vi "Set Direct Sampling.vi"(8 "error in (no error)":errorcluster, 10 "Direct Sampling State":T1, 11 "RTL-SDR in":refnum<class "RTL-SDR.lvclass">) -> (0 "error out":errorcluster, 1 "function return":i32, 3 "RTL-SDR out":refnum<class "RTL-SDR.lvclass">)   [LabVIEW 2015, in "RTL-SDR.lvclass"]
uses:
  RTL-SDR.lvclass
  TypeDef/Direct Sampling States.ctl
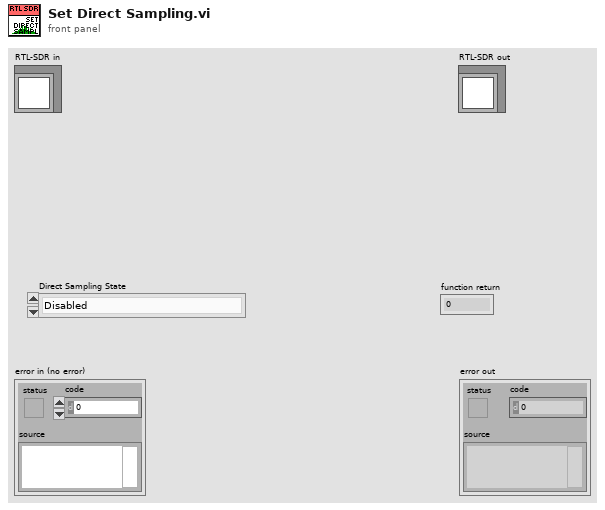
[diagram p1: front panel]
types:
  T1 = typedef "RTL-SDR.lvclass/Direct Sampling States.ctl" = enum16{"Disabled", "I-ADC Input Enabled", "Q-ADC Input Enabled"}
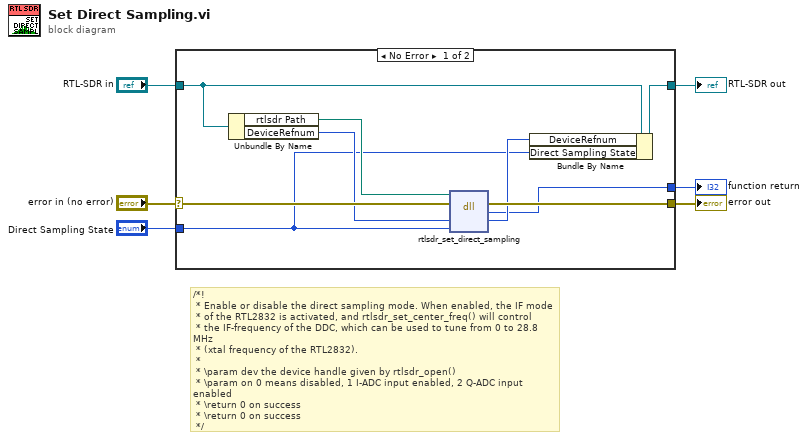
[diagram p0: block diagram]
diagram:
  # "/*!\n * Enable or disable the direct sampling mode. When enabled, the IF mode\n * of the RTL2832 is activated, and rtlsdr_set_center_freq() will control\n * the IF-frequency of the DDC, which can be used to tune from 0 to 28.8 MHz\n * (xtal frequency of the RTL2832).\n *\n * \\param dev the device handle given by rtlsdr_open()\n * \\param on 0 means disabled, 1 I-ADC input enabled, 2 Q-ADC input enabled\n * \\return 0 on success\n * \\return 0 on success\n */\n\n\nRTLSDR_API int rtlsdr_set_direct_sampling(rtlsdr_dev_t *dev, int on);"
  n1 = case shown="No Error" "error in (no error)" {
    selector: "error in (no error)" -> [w15 w17]
    tunnel: [w14 w17] -> w5
    tunnel: [w12 w16] -> w3
    tunnel: "RTL-SDR in" -> [w13 w16]
    tunnel: [w8 _] -> w2
    tunnel: "Direct Sampling State" -> [w7 _]
    frame No Error {
      n2 = Unbundle By Name(w13) -> ("rtlsdr Path"=w11:path, "DeviceRefnum"=w10:u64)
      n3 = dll-call lib="C:/Users/Ivan/Desktop/D-23-09-24 (RTL-SDR)/Project (Pelleng-SDR)/RTL-SDR Class/dll/rtlsdr.*" fn="rtlsdr_set_direct_sampling"(path in=w11, error in=w15, "DeviceRefnum"=w10, "Direct Sampling State"=w7) -> (error out=w14:errorcluster, "return type"=w8:i32, "DeviceRefnum"=w9:u64)  [unwired: 2 in, 1 out]
      n4 = Bundle By Name(cluster=w13, "DeviceRefnum"=w9, "Direct Sampling State"=w7) -> (w12:refnum<class "RTL-SDR.lvclass">)
    }
    frame Error {
    }
  }
  "error out" <- w5
  "RTL-SDR out" <- w3
  "function return" <- w2
